vi "Add User Channel_Channel and Folders.vi"(8 "error in (no error)":errorcluster, 9 "User Channel Settings":T1, 10 "Base Node Path":string, 11 "SysDef Ref":T2) -> (0 "error out":errorcluster, 3 "SysDef Ref Out":T2)   [LabVIEW 2019, in "Simple SysDef API.lvlib"]
uses:
  <userlib>/SimpleSysDef/Simple SysDef API.lvlib
  <userlib>/SimpleSysDef/_SubVIs/System Definition Reference.ctl
  NationalInstruments.VeriStand.SystemDefinitionAPI
  <userlib>/SimpleSysDef/_SubVIs/Add User Channel_Settings.ctl
  <userlib>/SimpleSysDef/_SubVIs/Add Folder_Settings.ctl
  <userlib>/SimpleSysDef/_SubVIs/Add User Channel Folder.vi
  <userlib>/SimpleSysDef/_SubVIs/Add User Channel.vi
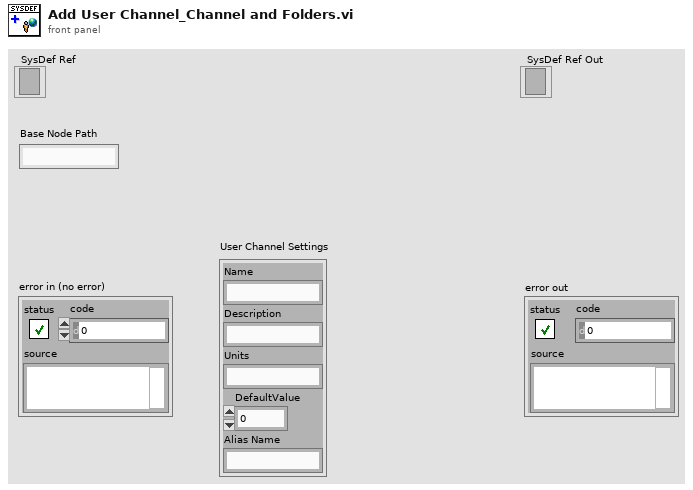
[diagram p1: front panel]
types:
  T1 = typedef "Simple SysDef API.lvlib/Add User Channel_Settings.ctl" = cluster{"Name":string, "Description":string, "Units":string, "DefaultValue":dbl, "Alias Name":string}
  T2 = typedef "Simple SysDef API.lvlib/System Definition Reference.ctl" = refnum<k24>
  T3 = typedef "Simple SysDef API.lvlib/Add Folder_Settings.ctl" = cluster{"Name":string, "Description":string}
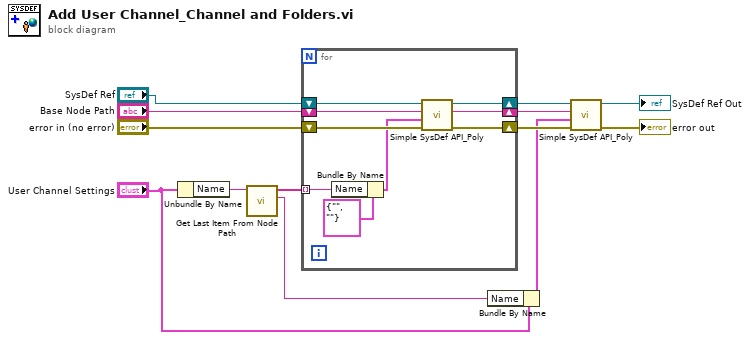
[diagram p0: block diagram]
diagram:
  n1 = Unbundle By Name("User Channel Settings") -> ("Name"=w5:string)
  n2 = call <userlib>:"Get Last Item From Node Path.vi"("Name"=w5) -> ("Last Item"=w2:string, "First Items"=w4:string[])  [unwired: 9 in]
  n3 = for {
    shift-right: [w21] -> w12
    shift-left: "error in (no error)" -> [w18]
    shift-right: [w20] -> w11
    shift-left: "Base Node Path" -> [w17]
    shift-right: [w22] -> w13
    shift-left: "SysDef Ref" -> [w19]
    tunnel: w4 -> [w16] mode=indexing
    n4 = Bundle By Name(cluster=T3 {"Name"="", "Description"=""} ("User Channel Folder Settings"), "Name"=w16) -> (w15:T3)
    n5 = call-poly <userlib>:"Simple SysDef API_Poly.vi"("error in (no error)"=w18, "User Channel Folder Settings"=w15, "Base Node Path"=w17, "SysDef Ref"=w19) -> ("error out"=w21:errorcluster, "New Node Path"=w20:string, "SysDef Ref Out"=w22:T2)  [unwired: 5 in]
  }
  n6 = Bundle By Name(cluster="User Channel Settings", "Name"=w2) -> (w1:T1)
  n7 = call-poly <userlib>:"Simple SysDef API_Poly.vi"("error in (no error)"=w12, "User Channel Settings"=w1, "Base Node Path"=w11, "SysDef Ref"=w13) -> ("error out"=→"error out":errorcluster, "SysDef Ref Out"=→"SysDef Ref Out":T2)  [unwired: 5 in, 1 out]
